vi "Change Num Coadd.vi"(8 "error in (no error)":errorcluster, 11 "tCRD in":refnum<class "tCRD.lvclass">) -> (0 "error out":errorcluster, 3 "tCRD out":refnum<class "tCRD.lvclass">)   [LabVIEW 2015, in "tCRD.lvclass"]
uses:
  tCRD.lvclass
  Reusable/CRDS/Main/CRDS.lvclass/CRDS.ctl
  Reusable/Instrument/Instrument.lvclass/Instrument.ctl
  Reusable/CRDS/Main/Write NumCoadd.vi
  Reusable/Instrument/Read Log Session.vi
  <userlib>/_Session Fwk/Session - Root.lvclass
  Reusable/Session Log/System Log.lvclass
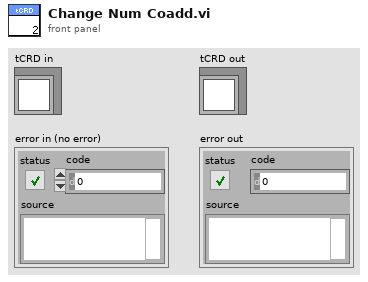
[diagram p1: front panel]
types:
  T1 = typedef "Session - Root.lvclass/Session Handle.ctl" = refnum<data-value>
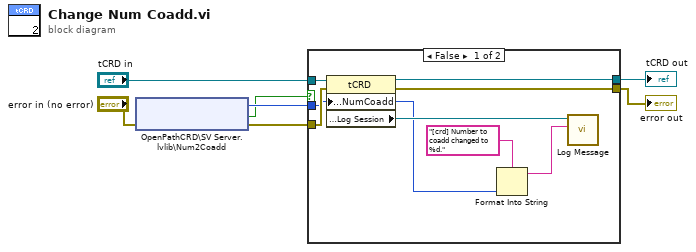
[diagram p0: block diagram]
diagram:
  n1 = shared-variable "OpenPathCRD\\SV Server.lvlib\\Num2Coadd"(error in="error in (no error)") -> (w5:u8, error out=w4:errorcluster, w3:bool)  [unwired: 1 in]
  n2 = case shown="False" w3 {
    tunnel: "tCRD in" -> [w15 w17]
    tunnel: [w14 w17] -> w6
    tunnel: w4 -> [w13 w16]
    tunnel: [w12 w16] -> w7
    tunnel: w5 -> [w10 _]
    frame False {
      n3 = property class="tCRD"(reference=w15, error in=w13, "Accessors:NumCoadd"=w10) -> (reference out=w14:refnum<class "tCRD.lvclass">, error out=w12:errorcluster, "Accessors:Log Session"=w11:T1)
      n4 = Format Into String(format string="[crd] Number to coadd changed to %d.", w10) -> (resulting string=w8:string)  [unwired: 2 in, 1 out]
      n5 = call "Log Message.vi"("MSG In"=w8, "session in"=w11) -> ()  [unwired: 8 in, 2 out]
    }
    frame True {
    }
  }
  "error out" <- w7
  "tCRD out" <- w6
